vi "USRP Dummy (FPGA).vi"() -> ()   [LabVIEW 2016]
uses:
  <instrlib>/_niInstr/Register Bus/v1/FPGA/Public/Read Cmd Data.ctl
  <vilib>/Platform/TimedLoop/XDataNode/timing_clust.ctl
  <vilib>/Platform/TimedLoop/XDataNode/nitl_modes.ctl
  <vilib>/Platform/TimedLoop/XDataNode/wakeup.ctl
  <vilib>/rvi/Emulation/niFpgaSctlEmulationGetInTimedLoop.vi
  <vilib>/rvi/Emulation/niFpgaEmulationReportErrorSimple.vi
  <vilib>/rvi/Emulation/niFpgaGetClockAttributes.vi
  <vilib>/rvi/Emulation/niFpgaCriticalErrorInLSC.vi
  <vilib>/rvi/eio/common/nirviEmuTemplateMethod_errors.vi
  <vilib>/rvi/interface/RandomDataEmulation/niFpgaRandomDataHandleErrors.vi
  <instrlib>/_niInstr/Basic Elements/v1/FPGA/Private/Count Up U64.vi
  <vilib>/Platform/TimedLoop/XDataNode/XDataNode.xnode
  <vilib>/eio/EIONode/EIONode.xnode
  <vilib>/rvi/DataTransferAndStorage/Container/XNode/niFpgaContainer.xnode
  <vilib>/rvi/interface/RandomDataEmulation/nirviRandomDataFpgaReadWriteTemplate.vi
  <vilib>/Platform/TimedLoop/XDataNode/XDNodeRunTimeDep.lvlib
  <instrlib>/_niInstr/Register Bus/v1/FPGA/niInstr Register Bus v1 FPGA.lvlib
  <instrlib>/niUsrpRio/Config/v1/FPGA/niUsrpRio Config v1 FPGA.lvlib
  <instrlib>/_niInstr/Basic Elements/v1/FPGA/niInstr Basic Elements v1 FPGA.lvlib
panel:
  out "Random Number":u64
  in  "Decimate (200MHz)":u32=2
  in  "Flush FIFO?":bool
  in  "Stop Transfer?":bool
  out "Min Space Available":u32
  out "Space Available":u32
  out "FPGA FIFO Depth":u32
  in  "Reset FPGA Count?":bool
  out "Samples Left to Write":u64
  in  "Number of Samples":u64
  in  "reg.host read.go rcvd 0":bool
  out "reg.notify host.go 0":bool
  in  "reg.notify host.go rcvd 0":bool
  out "reg.host read.data 0":T1
  in  "reg.reset 0":bool
  in  "RF 0/Rx/Enable":bool
  in  "RF 0/Tx/Enable":bool
  in  "RF 1/Rx/Enable":bool
  in  "RF 1/Tx/Enable":bool
  out "FPGA Count":u64
  in  "Start Transfer?":bool
  in  "Reset Timeouts?":bool
  out "Timeout Count":u64
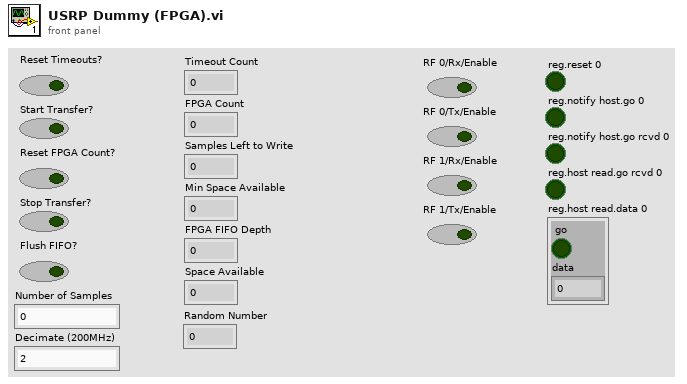
[diagram p1: front panel]
types:
  T1 = typedef "niInstr Register Bus v1 FPGA.lvlib/Read Cmd Data.ctl" = cluster{"go":bool, "data":u32}
  T2 = typedef "XDNodeRunTimeDep.lvlib/timing_clust.ctl" = cluster{"Expected End [f-1]":u64, "Actual End [f-1]":u64, "Finished Late? [f-1]":bool, "Expected End [i-1]":u64, "Actual End [i-1]":u64, "Finished Late? [i-1]":bool, "Expected Start [i]":u64, "Actual Start [i]":u64, "Expected Start [f]":u64, "Actual Start [f]":u64, "Source Name":string, "Structure Name":string, "Period":i64, "Deadline":i64, "Offset":i64, "Start":i64, "Priority":i32, "Timeout":i32, "Mode":T3, "Wakeup Reason":T4, "Error":errorcluster, "Source Type":string, "Secondary Source Type":string, "Global End Time":u64, "Global Start Time":u64, "Frame Duration":u64, "Iteration Duration":u64, "Assigned CPU":i32, "I/O Scan Engine Mode":u32}
  T3 = typedef "XDNodeRunTimeDep.lvlib/nitl_modes.ctl" = enum32{"No Change", "Process missed periods, maintain original phase", "Discard missed periods, maintain original phase", "Process missed periods, ignore original phase", "Discard missed periods, ignore original phase"}
  T4 = typedef "XDNodeRunTimeDep.lvlib/wakeup.ctl" = enum32{"Normal", "Aborted", "Asynchronous wakeup", "Timing source error", "Timed loop error", "Timeout"}
  T5 = cluster{"DAC FIFO Reset":refnum<k21>, "RF 0 Rx Swap IQ":refnum<k21>, "RF 0 Rx Negate I":refnum<k21>, "RF 0 Rx Negate Q":refnum<k21>, "RF 0 Rx Data Valid":refnum<k21>, "RF 0 Rx Data Ever Invalid":refnum<k21>, "clear RF 0 Rx Data Ever Invalid":refnum<k21>, "RF 0 Tx Swap IQ":refnum<k21>, "RF 0 Tx Negate I":refnum<k21>, "RF 0 Tx Negate Q":refnum<k21>, "RF 1 Rx Swap IQ":refnum<k21>, "RF 1 Rx Negate I":refnum<k21>, "RF 1 Rx Negate Q":refnum<k21>, "RF 1 Rx Data Valid":refnum<k21>, "RF 1 Rx Data Ever Invalid":refnum<k21>, "clear RF 1 Rx Data Ever Invalid":refnum<k21>, "RF 1 Tx Swap IQ":refnum<k21>, "RF 1 Tx Negate I":refnum<k21>, "RF 1 Tx Negate Q":refnum<k21>}
  T6 = typedef "niUsrpRio Synchronization v1 FPGA.lvlib/Resources.ctl" = cluster{"master":refnum<k21>, "meas.enable":refnum<k21>, "meas.ready":refnum<k21>, "meas.reset":refnum<k21>, "meas.arm":refnum<k21>, "meas.valid":refnum<k21>, "meas.value":refnum<k21>, "meas.oversample factor":refnum<k21>, "cptr":refnum<k21>, "cptr.adjust":refnum<k21>, "cptr.period":refnum<k21>}
  T7 = typedef "niUsrpRio Time v1 FPGA.lvlib/Time Resources.ctl" = cluster{"reset":refnum<k21>, "time":refnum<k21>, "time.previous cptr":refnum<k21>, "new time":refnum<k21>, "new time.when":refnum<k21>, "new time.set":refnum<k21>, "which edge of ref":refnum<k21>, "pps source":refnum<k21>, "internal pps period":refnum<k21>}
  T8 = typedef "niUsrpRio Time v1 FPGA.lvlib/Future Event Resources.ctl" = cluster{"reset":refnum<k21>, "future event.time":refnum<k21>, "future event.ready":refnum<k21>, "future event.set":refnum<k21>, "future event.clear":refnum<k21>, "future event.set in past":refnum<k21>}
  T9 = cluster{"time.resources":T7, "future event.resources":T8, "future event.resources":T8, "future event.resources":T8}
  T10 = typedef "niInstr Register Bus v1 FPGA.lvlib/Register Instruction.ctl" = cluster{"subsystem":u8, "address":u16, "data":u32, "valid":bool, "read":bool}
  T11 = typedef "niInstr Register Bus v1 FPGA.lvlib/Read Completion.ctl" = cluster{"data":u32, "valid":bool}
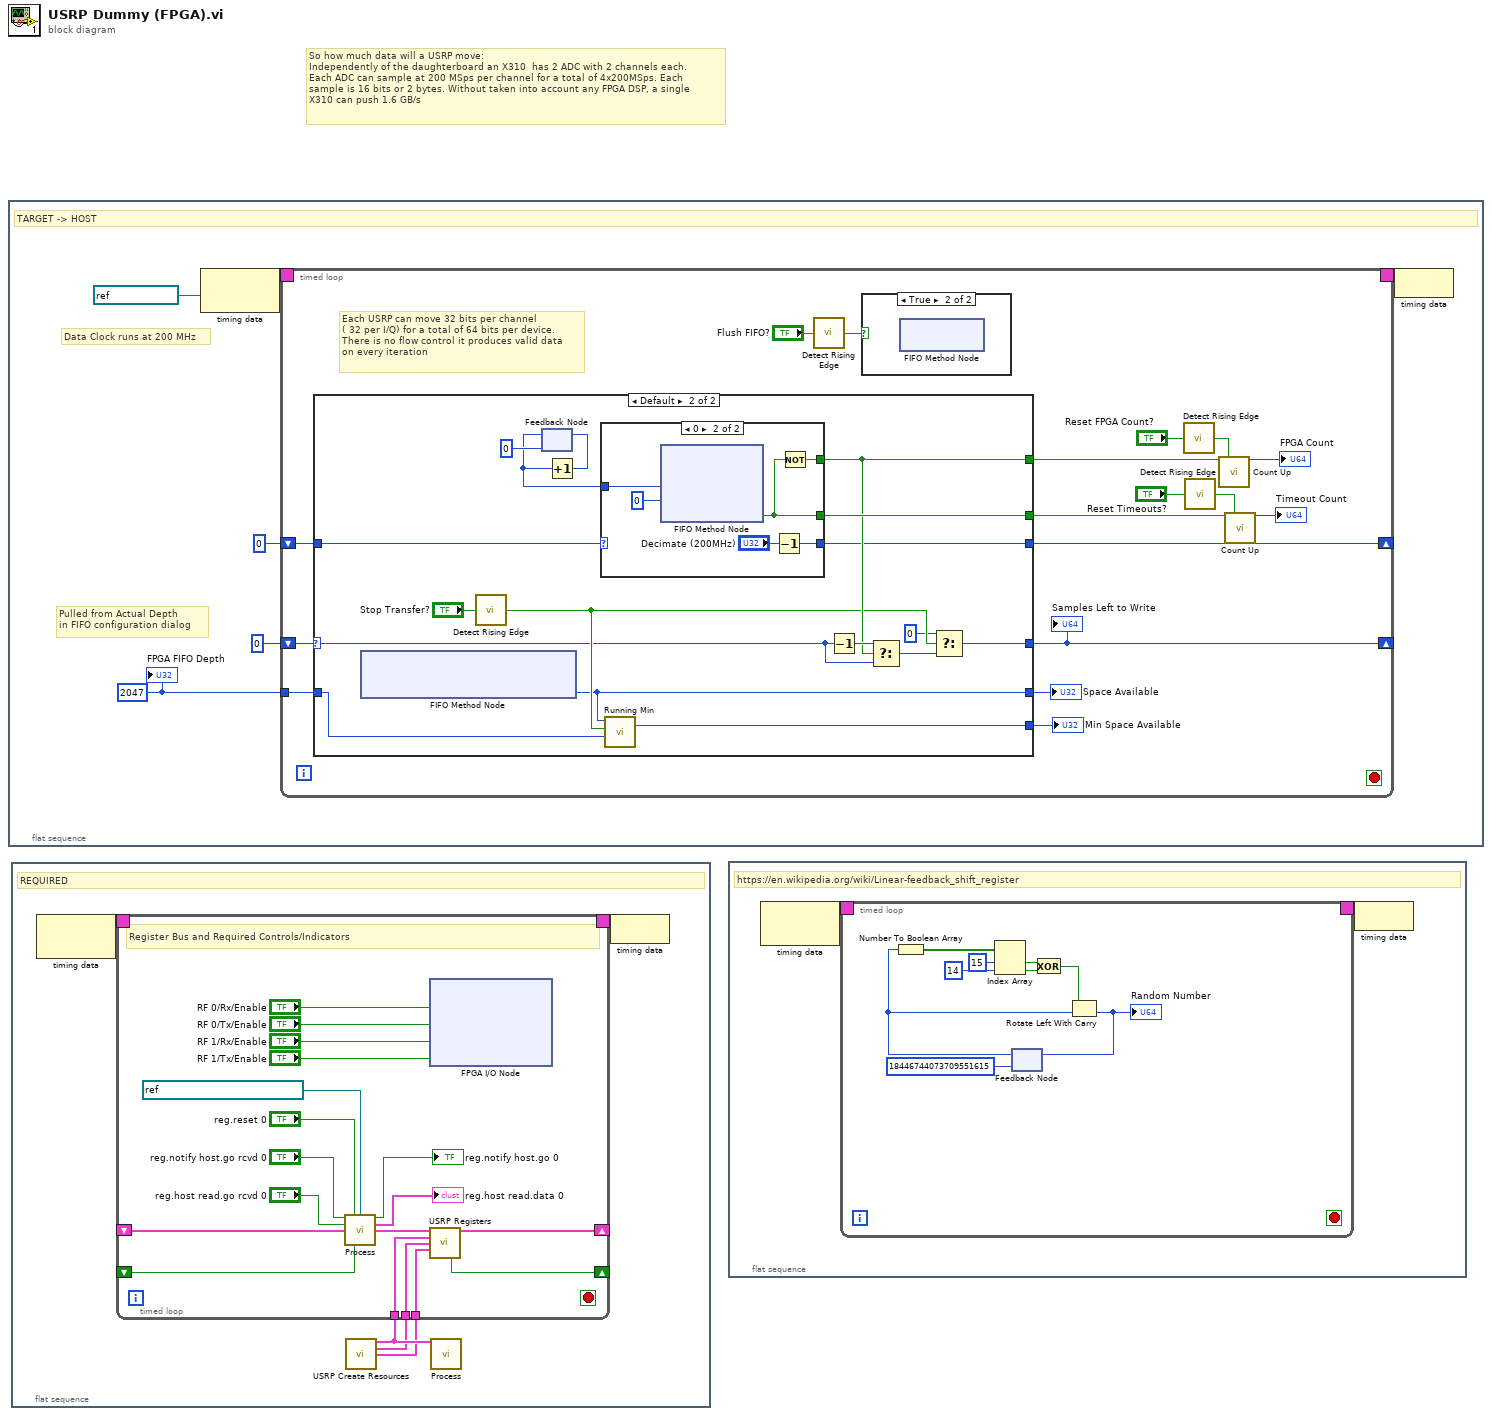
[diagram p0: block diagram]
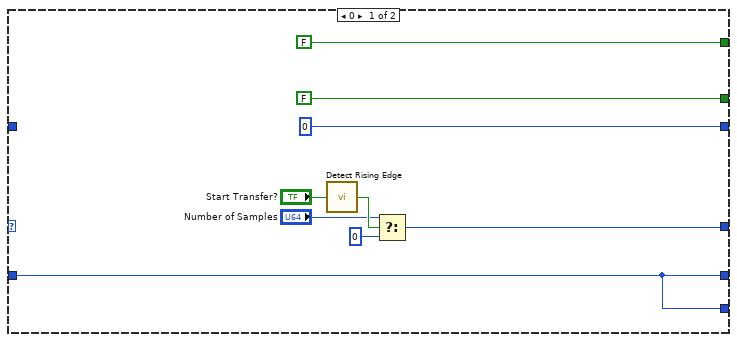
[diagram p3: hidden frame]
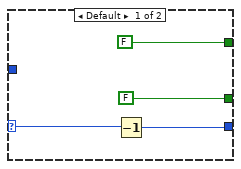
[diagram p4: hidden frame]
diagram:
  # "So how much data will a USRP move:\nIndependently of the daughterboard an X310  has 2 ADC with 2 channels each.\nEach ADC can sample at 200 MSps per channel for a total of 4x200MSps. Each \nsample is 16 bits or 2 bytes. Without taken into account any FPGA DSP, a single\nX310 can push 1.6 GB/s"
  n1 = flat-sequence {
    frame #0 {
      w2 = u32 2047 ("FPGA FIFO Depth")
      # "Pulled from Actual Depth\nin FIFO configuration dialog"
      # "Data Clock runs at 200 MHz"
      # "TARGET -> HOST"
      n2 = node-c288(refnum<k21> "Data Clock" ("Source Name")) -> (w6:T2)
      n3 = timed-loop {
        timing: w6 -> [_]
        timing-out: [_] -> w5
        shift-right: [w23] -> _
        shift-left: u64 0 ("samples to write") -> [w9]
        tunnel: w2 -> [w22]
        shift-right: [w15] -> _
        shift-left: u32 0 ("samples to write") -> [w14]
        stop <- _ stop-if-true
        # "Each USRP can move 32 bits per channel\n( 32 per I/Q) for a total of 64 bits per device.\nThere is no flow control it produces valid data\non every iteration"
        n4 = case shown="Default" w9 {
          selector: w9 -> [_ w39]
          tunnel: [FALSE ("Timed Out?") w45] -> w18
          tunnel: [FALSE ("Timed Out?") w46] -> w17
          tunnel: [w25 w37] -> w23
          tunnel: w22 -> [w24 w48]
          tunnel: [u32 0 w40] -> w15
          tunnel: w14 -> [_ w41]
          tunnel: [w24 w34] -> w8
          tunnel: [w24 w33] -> w7
          frame 0 {
            n5 = call <instrlib>:"Detect Rising Edge.vi"("signal"="Start Transfer?") -> ("edge detected"=w28:bool)  [unwired: 14 in]
            n6 = Select(t="Number of Samples", s=w28, f=u64 0) -> (s? t:f=w25:u64)
          }
          frame Default {
            n7 = xnode ("FIFO Method Node")() -> ("Number of Elements to Write"=w34:u32)  [unwired: 1 in, 1 out]
            n8 = call <instrlib>:"Detect Rising Edge.vi"("signal"="Stop Transfer?") -> ("edge detected"=w42:bool)  [unwired: 14 in]
            n9 = feedback #1(u64 0) -> (w35:u64)
            n10 = Increment(x=w35) -> (x+1=w43:u64)
            n11 = feedback-in #1(w43) -> ()
            n12 = case shown="0" w41 {
              selector: w41 -> [w51 _]
              tunnel: w35 -> [_ w59]
              tunnel: [FALSE ("Timed Out?") w58] -> w46
              tunnel: [FALSE ("Timed Out?") w57] -> w45
              tunnel: [w50 w54] -> w40
              frame Default {
                n13 = Decrement(x=w51) -> (x-1=w50:u32)
              }
              frame 0 {
                n14 = xnode ("FIFO Method Node")("Element"=w59, "Timeout"=0) -> ("Timed Out?"=w58:bool)  [unwired: 1 in, 1 out]
                n15 = Decrement(x="Decimate (200MHz)") -> (x-1=w54:u32)
                n16 = Not(x=w58) -> (.not. x?=w57:bool)
              }
            }
            n17 = call "Running Min.vi"("Starting Min"=w48, "Reset"=w42, "Next Value"=w34) -> ("Running Min"=w33:u32)  [unwired: 4 in]
            n18 = Decrement(x=w39) -> (x-1=w49:u64)
            n19 = Select(t=w49, s=w45, f=w39) -> (s? t:f=w38:u64)
            n20 = Select(t=u64 0, s=w42, f=w38) -> (s? t:f=w37:u64)
          }
        }
        "Samples Left to Write" <- w23
        "Space Available" <- w8
        "Min Space Available" <- w7
        n21 = call <instrlib>:"Detect Rising Edge.vi"("signal"="Flush FIFO?") -> ("edge detected"=w20:bool)  [unwired: 14 in]
        n22 = case shown="True" w20 {
          frame False {
          }
          frame True {
            n23 = xnode ("FIFO Method Node")() -> ()  [unwired: 1 in, 1 out]
          }
        }
        n24 = call <instrlib>:"Detect Rising Edge.vi"("signal"="Reset FPGA Count?") -> ("edge detected"=w12:bool)  [unwired: 14 in]
        n25 = call <instrlib>:"Detect Rising Edge.vi"("signal"="Reset Timeouts?") -> ("edge detected"=w10:bool)  [unwired: 14 in]
        n26 = call-poly <instrlib>:"Count Up.vi"("increment"=w18, "reset"=w12) -> ("count out"=→"FPGA Count":u64)  [unwired: 13 in]
        n27 = call-poly <instrlib>:"Count Up.vi"("increment"=w17, "reset"=w10) -> ("count out"=→"Timeout Count":u64)  [unwired: 13 in]
      }
      n28 = node-c288(w5) -> ()
      "FPGA FIFO Depth" <- w2
    }
  }
  n29 = flat-sequence {
    frame #0 {
      # "REQUIRED"
      n30 = node-c288() -> (w70:T2)  [unwired: 1 in]
      n31 = call "USRP Create Resources.vi"() -> ("config.resources"=w68:T5, "sync.resources"=w67:T6, "time.resources"=w66:T9)  [unwired: 13 in]
      n32 = timed-loop "Register Bus and Required Controls/Indicators" {
        timing: w70 -> [_]
        timing-out: [_] -> w69
        shift-right: [w85] -> _
        shift-left: _ -> [w84]
        shift-right: [w79] -> _
        shift-left: _ -> [w83]
        tunnel: w68 -> [w77]
        tunnel: w67 -> [w76]
        tunnel: w66 -> [w75]
        stop <- _ stop-if-true
        # "Register Bus and Required Controls/Indicators"
        n33 = call <instrlib>:"Process.vi"("reg.notify host.go rcvd"="reg.notify host.go rcvd 0", "reg.reset"="reg.reset 0", "reg.host instruction fifo"=refnum<k21> "reg.host instruction fifo 0", "reg.host read.go rcvd"="reg.host read.go rcvd 0", "read completion"=w84, "ready for output"=w83) -> ("reg.notify host.go"=→"reg.notify host.go 0":bool, "reg.host read.data"=→"reg.host read.data 0":T1, "register instruction"=w78:T10)  [unwired: 7 in]
        n34 = xnode ("FPGA I/O Node")("RF 0/Rx/Enable"="RF 0/Rx/Enable", "RF 0/Tx/Enable"="RF 0/Tx/Enable", "RF 1/Rx/Enable"="RF 1/Rx/Enable", "RF 1/Tx/Enable"="RF 1/Tx/Enable") -> ()  [unwired: 4 in, 4 out]
        n35 = call "USRP Registers.vi"("register instruction"=w78, "config.resources"=w77, "sync.resources"=w76, "time.resources"=w75) -> ("read completion out"=w85:T11, "ready for input"=w79:bool)  [unwired: 10 in]
      }
      n36 = call <instrlib>:"Process.vi"("resources"=w68) -> ()  [unwired: 15 in]
      n37 = node-c288(w69) -> ()
    }
  }
  n38 = flat-sequence {
    frame #0 {
      # "https://en.wikipedia.org/wiki/Linear-feedback_shift_register"
      n39 = node-c288() -> (w94:T2)  [unwired: 1 in]
      n40 = timed-loop {
        timing: w94 -> [_]
        timing-out: [_] -> w93
        stop <- _ stop-if-true
        n41 = feedback #2(u64 18446744073709551615) -> (w97:u64)
        n42 = Number To Boolean Array(number=w97) -> (Boolean array=w103:bool[])
        n43 = Index Array(array=w103, index #1=15 ("index"), index #2=14 ("index")) -> (element #1=w99:bool, element #2=w98:bool)
        n44 = Exclusive Or(1:w98, 2:w99) -> (0:w96:bool)
        n45 = Rotate Left With Carry(2:w97, 3:w96) -> (0:w95:u64)  [unwired: 1 out]
        "Random Number" <- w95
        n46 = feedback-in #2(w95) -> ()
      }
      n47 = node-c288(w93) -> ()
    }
  }
